vi "InitDone.vi"(8 "error in (no error)":errorcluster, 10 "Variant":variant, 11 "SpectrumAnalyzerUI.lvclass":refnum<class "SpectrumAnalyzerUI.lvclass">) -> (0 "error out":errorcluster, 3 "SpectrumAnalyzerUI.lvclass":refnum<class "SpectrumAnalyzerUI.lvclass">)   [LabVIEW 2023, in "SpectrumAnalyzerUI.lvlib" / "SpectrumAnalyzerUI.lvclass"]
uses:
  SpectrumAnalyzerUI.lvclass
  SpectrumAnalyzerUI.lvclass/SpectrumAnalyzerUI.ctl
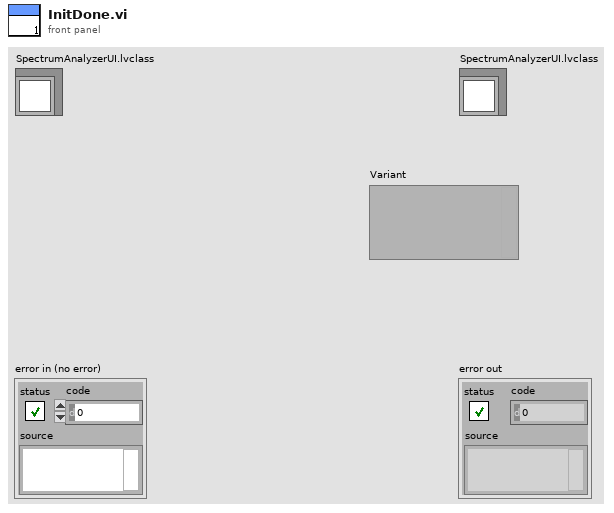
[diagram p1: front panel]
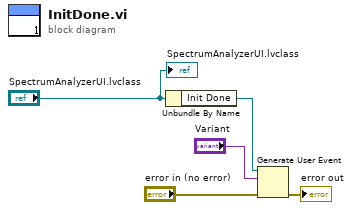
[diagram p0: block diagram]
diagram:
  n1 = Unbundle By Name("SpectrumAnalyzerUI.lvclass") -> ("Init Done"=w4:refnum<user-event>)
  n2 = Generate User Event(user event=w4, event data cluster="Variant", error in="error in (no error)") -> (error out=→"error out":errorcluster)  [unwired: 1 in, 1 out]
  "SpectrumAnalyzerUI.lvclass" <- "SpectrumAnalyzerUI.lvclass"
